vi "LCD Init.vi"(8 "error in":errorcluster, 11 "FPGA VI Reference in":T3) -> (0 "error out":errorcluster, 3 "FPGA VI Reference Out":T3)   [LabVIEW 2019]
uses:
  TypeDefs/FPGA Reference.ctl
  TypeDefs/Line.ctl
  TypeDefs/Pixel.ctl
  TypeDefs/Type of message.ctl
panel:
  in  "stop 2":bool
  in  "Line":T1={"Start"={"X0"=0, "Y0"=0}, "end"={"X0"=320, "Y0"=0}}
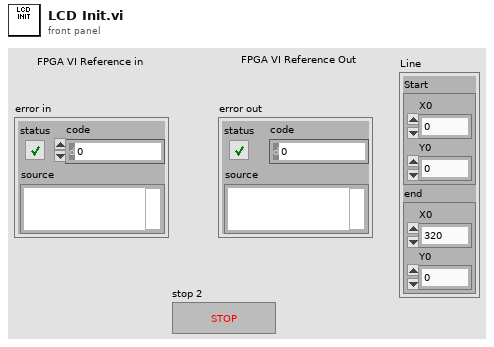
[diagram p1: front panel]
types:
  T1 = typedef "Line.ctl" = cluster{"Start":T2, "end":T2}
  T2 = typedef "Pixel.ctl" = cluster{"X0":i16, "Y0":i16}
  T3 = typedef "FPGA Reference.ctl" = refnum<k20>
  T4 = typedef "Type of message.ctl" = enum16{"CMD", "DATA"}
  T5 = typedef "imagedata.ctl" = cluster{"image type":i32, "image depth":i32, "image":u8[], "mask":u8[], "colors":u32[], "Rectangle":cluster{"left":i16, "top":i16, "right":i16, "bottom":i16}}
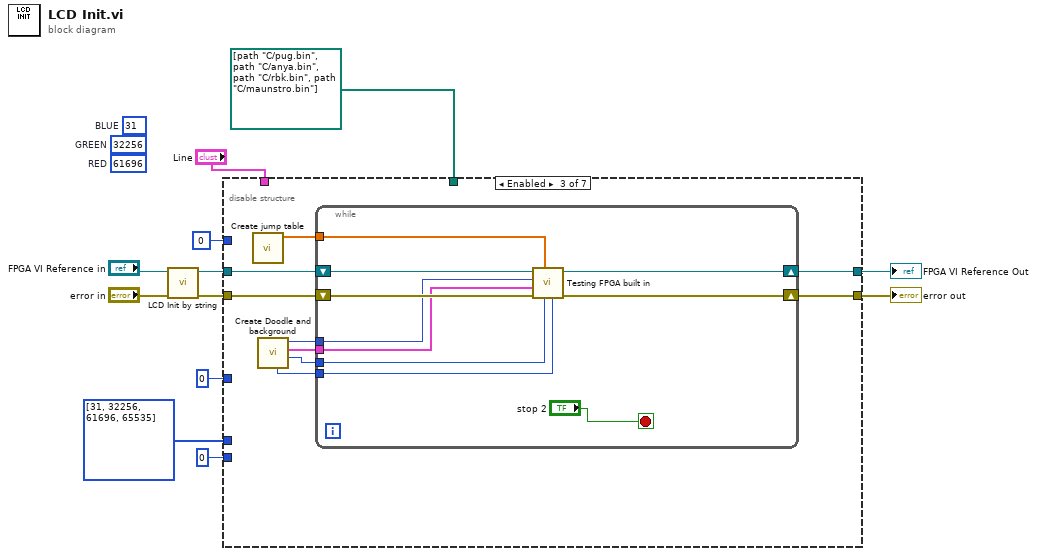
[diagram p0: block diagram]
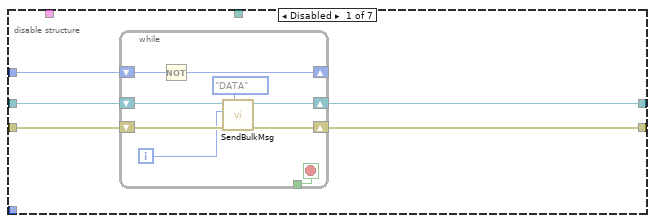
[diagram p2: hidden frame]
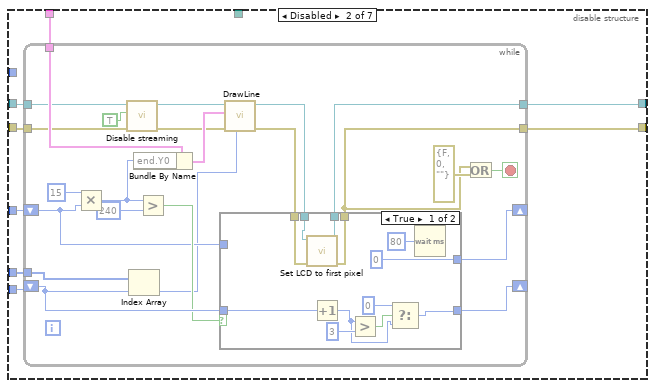
[diagram p3: hidden frame]
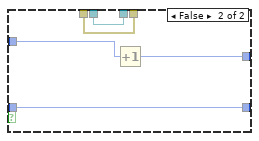
[diagram p4: hidden frame]
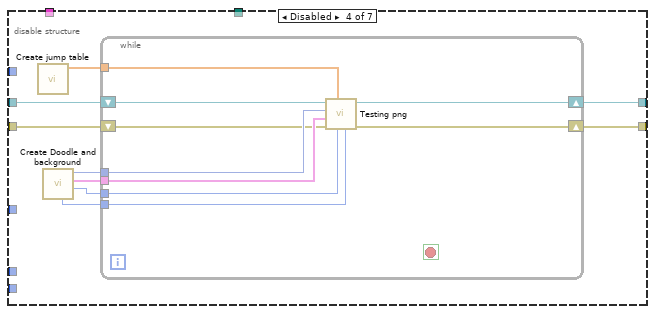
[diagram p5: hidden frame]
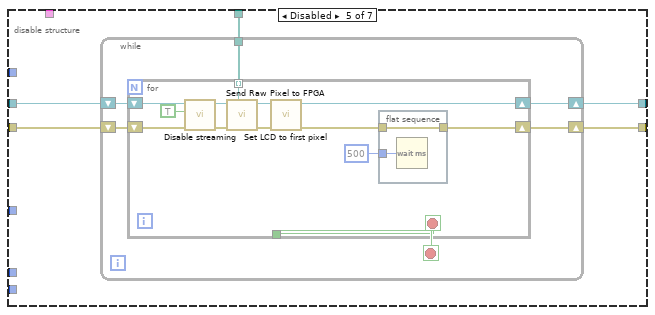
[diagram p6: hidden frame]
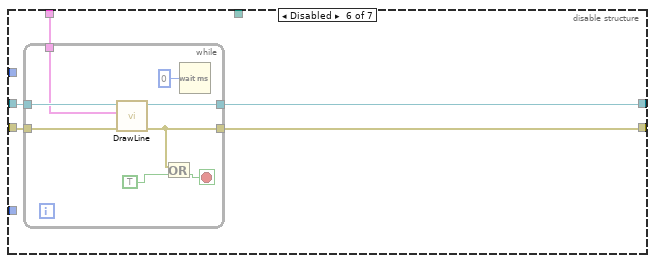
[diagram p7: hidden frame]
diagram:
  (unwired) u16 32256  # GREEN
  (unwired) u16 61696  # RED
  (unwired) u16 31  # BLUE
  n1 = call "LCD Init by string.vi"("error in"="error in", "FPGA VI Reference In"="FPGA VI Reference in") -> ("error out"=w9:errorcluster, "FPGA VI Reference Out"=w11:T3)  [unwired: 8 in]
  n2 = disable-structure shown="Enabled" {
    disable-tunnel: [w18 w32 w81 w100 w114 w140 w152] -> w12
    disable-tunnel: w11 -> [w17 w35 w84 w103 w117 w143 w153]
    disable-tunnel: u16 0 ("Payload") -> [w16 _ _ _ _ _ _]
    disable-tunnel: w9 -> [w15 w33 w83 w102 w116 w141 w152]
    disable-tunnel: [w14 w34 w82 w101 w115 w142 w153] -> w8
    disable-tunnel: "Line" -> [_ w31 _ _ _ w139 _]
    disable-tunnel: u16[] [31, 32256, 61696, 65535] -> [_ w30 _ _ _ _ _]
    disable-tunnel: 0 ("index") -> [_ w29 _ _ _ _ _]
    disable-tunnel: 0 ("index") -> [_ w28 _ _ _ _ _]
    disable-tunnel: path[] [path "C:/pug.bin", path "C:/anya.bin", path "C:/rbk.bin", path "C:/maunstro.bin"] -> [_ _ _ _ w113 _ _]
    frame Disabled {
      n3 = while {
        shift-right: [w24] -> w18
        shift-left: w15 -> [w27]
        shift-right: [w25] -> w14
        shift-left: w17 -> [w26]
        shift-right: [w22] -> _
        shift-left: w16 -> [w21]
        tunnel: [w19] -> w13
        i -> [w20]
        stop <- w19 stop-if-true
        n4 = Not(x=w21) -> (.not. x?=w22:u16)
        n5 = call "SendBulkMsg.vi"("MsgType"=Type_of_message."DATA", "error in"=w27, "Payload"=w20, "FPGA VI Reference In"=w26) -> ("error out"=w24:errorcluster, "FPGA VI Reference Out"=w25:T3)  [unwired: 6 in]
      }
    }
    frame Disabled {
      n6 = while {
        tunnel: w35 -> [w43]
        tunnel: [w37] -> w34
        tunnel: w33 -> [w44]
        tunnel: [w38] -> w32
        tunnel: w31 -> [w57]
        tunnel: w30 -> [w53]
        shift-right: [w51] -> _
        shift-left: w29 -> [w52]
        shift-right: [w48] -> _
        shift-left: w28 -> [w49]
        stop <- w47 stop-if-true
        n7 = Multiply(x=15, y=w49) -> (x*y=w55:i32)
        n8 = call "Disable streaming.vi"("error in"=w44, "StreamDisabled"=TRUE, "FPGA VI Reference Out"=w43) -> ("error out"=w41:errorcluster, "FPGA VI Reference Out 2"=w42:T3)  [unwired: 7 in]
        n9 = Index Array(array=w53, index=w52) -> (element=w36:u16)
        n10 = Bundle By Name(cluster=w57, "end.Y0"=w55) -> (w56:T1)
        n11 = Greater?(x=w55, y=240) -> (0:w50:bool)
        n12 = call "DrawLine.vi"("Color"=w36, "error in"=w41, "Line"=w56, "FPGA VI Reference In"=w42) -> ("error out"=w40:errorcluster, "FPGA VI Reference Out"=w39:T3)  [unwired: 6 in]
        n13 = case shown="True" w50 {
          tunnel: w52 -> [w70 w75]
          tunnel: [w64 w75] -> w51
          tunnel: w49 -> [_ w74]
          tunnel: [0 w73] -> w48
          tunnel: w40 -> [w63 w71]
          tunnel: w39 -> [w62 w72]
          tunnel: [w61 w71] -> w38
          tunnel: [w60 w72] -> w37
          frame True {
            n14 = call "Set LCD to first pixel.vi"("error in"=w63, "FPGA VI Reference In"=w62) -> ("error out"=w61:errorcluster, "FPGA VI Reference Out"=w60:T3)  [unwired: 8 in]
            n15 = Increment(x=w70) -> (x+1=w65:i32)
            n16 = Greater?(x=w65, y=3) -> (0:w67:bool)
            n17 = Select(t=0, s=w67, f=w65) -> (s? t:f=w64:i32)
            n18 = Wait (ms)(milliseconds to wait=u32 80) -> ()  [unwired: 1 out]
          }
          frame False {
            n19 = Increment(x=w74) -> (x+1=w73:i32)
          }
        }
        n20 = Or(x=w38, y=errorcluster {"status"=FALSE, "code"=0, "source"=""}) -> (x .or. y?=w47:bool)
      }
    }
    frame Enabled {
      n21 = call "Create jump table.vi"() -> ("Array"=w80:dbl[])  [unwired: 11 in]
      n22 = call "Create Doodle and background.vi"() -> ("top"=w77:i16, "Doodle out"=w79:T5, "background"=w78:picture, "bottom"=w76:i16)  [unwired: 8 in]
      n23 = while {
        shift-right: [w85] -> w82
        shift-left: w84 -> [w93]
        shift-right: [w86] -> w81
        shift-left: w83 -> [w92]
        tunnel: w80 -> [w91]
        tunnel: w79 -> [w89]
        tunnel: w78 -> [w90]
        tunnel: w77 -> [w88]
        tunnel: w76 -> [w87]
        stop <- "stop 2" stop-if-true
        n24 = call "Testing FPGA built in.vi"("bottom"=w87, "top"=w88, "Jump Table"=w91, "error in"=w92, "Doodle in"=w89, "background"=w90, "FPGA VI Reference In"=w93) -> ("error out"=w86:errorcluster, "FPGA VI Reference Out"=w85:T3)  [unwired: 3 in]
      }
    }
    frame Disabled {
      n25 = call "Create jump table.vi"() -> ("Array"=w99:dbl[])  [unwired: 11 in]
      n26 = call "Create Doodle and background.vi"() -> ("top"=w96:i16, "Doodle out"=w98:T5, "background"=w97:picture, "bottom"=w95:i16)  [unwired: 8 in]
      n27 = while {
        shift-right: [w104] -> w101
        shift-left: w103 -> [w105]
        shift-right: [w107] -> w100
        shift-left: w102 -> [w106]
        tunnel: w99 -> [w112]
        tunnel: w98 -> [w111]
        tunnel: w97 -> [w110]
        tunnel: w96 -> [w109]
        tunnel: w95 -> [w108]
        stop <- _ stop-if-true
        n28 = call "Testing png.vi"("bottom"=w108, "top"=w109, "Jump Table"=w112, "error in"=w106, "Doodle in"=w111, "background"=w110, "FPGA VI Reference In"=w105) -> ("error out"=w107:errorcluster, "FPGA VI Reference Out"=w104:T3)  [unwired: 3 in]
      }
    }
    frame Disabled {
      n29 = while {
        shift-right: [w121] -> w115
        shift-left: w117 -> [w123]
        shift-right: [w120] -> w114
        shift-left: w116 -> [w122]
        tunnel: w113 -> [w119]
        stop <- w118 stop-if-true
        n30 = for {
          tunnel: w119 -> [w136] mode=indexing
          shift-right: [w127] -> w121
          shift-left: w123 -> [w135]
          shift-right: [w124] -> w120
          shift-left: w122 -> [w134]
          tunnel: [w130] -> w118
          stop <- w130 stop-if-true
          n31 = call "Disable streaming.vi"("error in"=w134, "StreamDisabled"=TRUE, "FPGA VI Reference Out"=w135) -> ("error out"=w133:errorcluster, "FPGA VI Reference Out 2"=w132:T3)  [unwired: 7 in]
          n32 = call "Send Raw Pixel to FPGA.vi"("file path (use dialog)"=w136, "error in"=w133, "FPGA VI Reference Out"=w132) -> ("error out"=w129:errorcluster, "FPGA VI Reference Out 2"=w128:T3)  [unwired: 7 in]
          n33 = call "Set LCD to first pixel.vi"("error in"=w129, "FPGA VI Reference In"=w128) -> ("error out"=w125:errorcluster, "FPGA VI Reference Out"=w127:T3)  [unwired: 8 in]
          n34 = flat-sequence {
            tunnel: u32 500 -> [w138]
            tunnel: w125 -> [w137]
            tunnel: [w137] -> w124
            frame #0 {
              n35 = Wait (ms)(milliseconds to wait=w138) -> ()  [unwired: 1 out]
            }
          }
        }
      }
    }
    frame Disabled {
      n36 = while {
        tunnel: w143 -> [w151]
        tunnel: [w150] -> w142
        tunnel: w141 -> [w148]
        tunnel: [w146] -> w140
        tunnel: w139 -> [w145]
        stop <- w147 stop-if-true
        n37 = call "DrawLine.vi"("error in"=w148, "Line"=w145, "FPGA VI Reference In"=w151) -> ("error out"=w146:errorcluster, "FPGA VI Reference Out"=w150:T3)  [unwired: 7 in]
        n38 = Or(x=w146, y=TRUE) -> (x .or. y?=w147:bool)
        n39 = Wait (ms)(milliseconds to wait=u32 0) -> ()  [unwired: 1 out]
      }
    }
    frame Disabled {
    }
  }
  "error out" <- w12
  "FPGA VI Reference Out" <- w8
